vi "FalseColor.vi"(2 "Image":T2, 3 "maxValue":dbl=4095.0, 4 "Operator":T1(ring)=enum."Clear  if > or =", 5 "error in (no error)":errorcluster) -> (22 "Image Dst Out":T2, 25 "error out":errorcluster)   [LabVIEW 2016]
uses:
  <vilib>/vision/Image Controls.llb/IMAQ Image.ctl
  <vilib>/vision/NI_Vision_Development_Module.lvlib
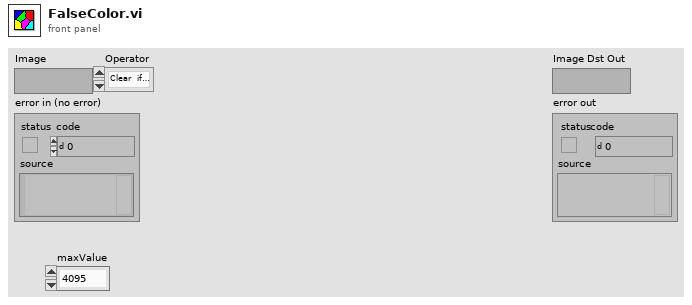
[diagram p1: front panel]
types:
  T1 = enum32{"Average", "Min", "Max", "Clear  if < ", "Clear  if < or =", "Clear  if =", "Clear  if > or =", "Clear  if >"}
  T2 = typedef "IMAQ Image.ctl" = refnum<image>
  T3 = enum32{"Gray", "Binary", "Gradient", "Rainbow", "Temperature"}
  T4 = typedef "Image Type" = u32
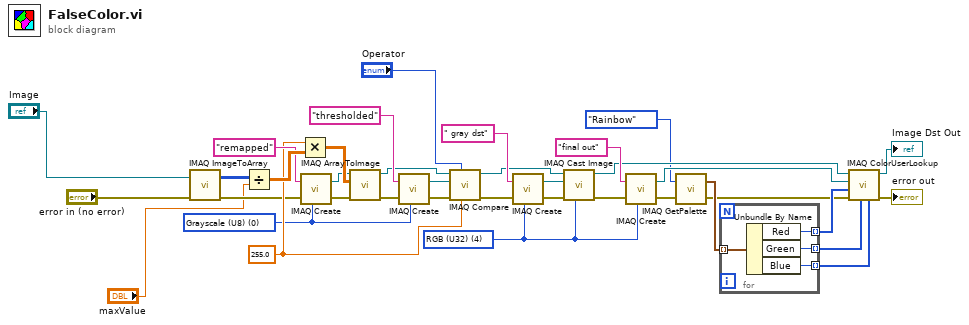
[diagram p0: block diagram]
diagram:
  w3 = T4 0 items=["Grayscale (U8)", "Grayscale (I16)", "Grayscale (SGL)", "Complex (CSG)", "RGB (U32)", "HSL (U32)", "RGB (U64)", "Grayscale (U16)"] ("Image Type")
  w20 = 255.0 ("x")
  w19 = T4 4 items=["Grayscale (U8)", "Grayscale (I16)", "Grayscale (SGL)", "Complex (CSG)", "RGB (U32)", "HSL (U32)", "RGB (U64)", "Grayscale (U16)"] ("Image Type")
  n1 = call "IMAQ ImageToArray"("error in (no error)"="error in (no error)", "Image"="Image") -> ("error out"=w5:errorcluster, "Image Pixels (I16)"=w1:i16[][])  [unwired: 2 in, 3 out]
  n2 = Divide(x=w1, y="maxValue") -> (x/y=w28:dbl[][])
  n3 = Multiply(x=w20, y=w28) -> (x*y=w27:dbl[][])
  n4 = call "IMAQ Create"("Image Name"="remapped", "Image Type"=w3, "error in (no error)"=w5) -> ("New Image"=w25:T2, "error out"=w15:errorcluster)  [unwired: 2 in]
  n5 = call "IMAQ ArrayToImage"("error in (no error)"=w15, "Image Pixels (U8)"=w27, "Image"=w25) -> ("error out"=w14:errorcluster, "Image Out"=w21:T2)  [unwired: 7 in]
  n6 = call "IMAQ Create"("Image Name"="thresholded", "Image Type"=w3, "error in (no error)"=w14) -> ("New Image"=w23:T2, "error out"=w13:errorcluster)  [unwired: 2 in]
  n7 = call "IMAQ Compare"("Constant"=w20, "Operator"="Operator", "error in (no error)"=w13, "Image Dst"=w23, "Image Src A"=w21) -> ("error out"=w12:errorcluster, "Image Dst Out"=w22:T2)  [unwired: 5 in]
  n8 = call "IMAQ Create"("Image Name"=" gray dst", "Image Type"=w19, "error in (no error)"=w12) -> ("New Image"=w31:T2, "error out"=w11:errorcluster)  [unwired: 1 in, 1 out]
  n9 = call "IMAQ Cast Image"("Image Type"=w19, "error in (no error)"=w11, "Image Dst"=w31, "Image Src"=w22) -> ("error out"=w10:errorcluster, "Image Dst Out"=w29:T2)  [unwired: 6 in]
  n10 = call "IMAQ Create"("Image Name"="final out", "Image Type"=w19, "error in (no error)"=w10) -> ("New Image"=w37:T2, "error out"=w9:errorcluster)  [unwired: 2 in]
  n11 = call "IMAQ GetPalette"("Palette Number (gray)"=T3."Rainbow", "error in (no error)"=w9) -> ("Color Palette"=w33:cluster{"Red":u8, "Green":u8, "Blue":u8}[], "error out"=w8:errorcluster)  [unwired: 3 in]
  n12 = for {
    tunnel: w33 -> [w41] mode=indexing
    tunnel: [w40] -> w34 mode=indexing
    tunnel: [w39] -> w35 mode=indexing
    tunnel: [w38] -> w36 mode=indexing
    n13 = Unbundle By Name(w41) -> ("Red"=w40:u8, "Green"=w39:u8, "Blue"=w38:u8)
  }
  n14 = call "IMAQ ColorUserLookup"("Blue or Luma or Val or Inten Lookup Table"=w36, "Green or Sat Lookup Table"=w35, "error in (no error)"=w8, "Red or Hue Lookup Table"=w34, "Image Dst"=w37, "Image Src"=w29) -> ("error out"=→"error out":errorcluster, "Image Dst Out"=→"Image Dst Out":T2)  [unwired: 4 in]
